vi "MenuToolOptions__slk_mt.vi"() -> ()   [LabVIEW 2020, in "Lazyboots Menu Tool.lvlib"]
uses:
  Library/Lazyboots Menu Tool.lvlib
  Private/Options/TypeDef/TypeDef_ParentSymbol__slk_mt.ctl
  Private/Options/TypeDef/TypeDef_MenuToolList__slk_mt.ctl
  Private/Options/TypeDef/TypeDef_FrameWidth__slk_mt.ctl
  Private/Options/TypeDef/TypeDef_FPGridSize.ctl
  Private/Options/TypeDef/TypeDef_ConnectorPattern__slk_mt.ctl
  Private/Options/TypeDef/TypeDef_ErrorControlStyle__slk_mt.ctl
  Private/Options/TypeDef/TypeDef_ErrorStyle__slk_mt.ctl
  Private/Options/TypeDef/TypeDef_PanelPosition__slk_mt.ctl
  Private/Options/TypeDef/TypeDef_ControlLabelPosition__slk_mt.ctl
  Private/Options/TypeDef/TypeDef_IndicatorLabelPosition__slk_mt.ctl
  Private/Options/TypeDef/TypeDef_ControlStyle__slk_mt.ctl
  Private/Options/Class/GUI/GUI__slk_mt.lvclass
  <vilib>/Utility/config.llb/NI_LVConfig.lvlib
panel:
  in  "Button: Restore":bool
  in  "Button: Cancel":bool
  in  "Button: OK":bool
  in  "Menu Tool Options":T1(tab)
  in  "Resize Panel: Ignore Decorations":bool
  in  "Resize Panel: Set Block Diagram":bool=TRUE
  in  "Resize Panel: BD Frame Width":T2=24 caption="Frame Width (pixels)"
  in  "Resize Panel: Ignore Hidden":bool=TRUE
  in  "Resize Panel: FP Position":T3="Top Left" caption="Position"
  in  "Resize Panel: FP Frame Width":T2=24 caption="Frame Width (pixels)"
  in  "Resize Panel: Set Origin":bool=TRUE
  in  "Resize Panel: Set Front Panel":bool=TRUE
  in  "Set Label Position: Apply to All":bool
  in  "Set Label Position: Indicator Label Position":T4="Right Middle" caption="Indicator Label Position"
  in  "Set Label Position: Control Label Position":T5="Left Middle" caption="Control Label Position"
  in  "Add Error: Snap to Grid":bool=TRUE
  in  "Add Error: FP Grid Size":T6=12 caption="FP Grid Size  (pixels)"
  in  "Add Error: Error Style":T7="2 Columns Style" caption="Error Style"
  in  "Add Error: Control Style":T8="Classic Style" caption="Control Style"
  in  "Add Error: Connector Pattern":T9=4815 caption="Connector Pattern" items=["4801"=4801, "4805"=4805, "4810"=4810, "4812"=4812, "4815"=4815, "4820"=4820, "4826"=4826, "4833"=4833, "4834"=4834, "4835"=4835]
  in  "Add Error: Wire to Connector":bool=TRUE
  in  "Add Error: Frame Width":T2=24 caption="Frame Width  (pixels)"
  in  "Add Error Case: Frame Width":T2=24 caption="Frame Width (pixels)"
  in  "Add Error Case: Create Constant":bool=TRUE
  in  "Create Enum: Control Style":T10="Classic Style" caption="Control Style"
  in  "Create Enum: New":bool=TRUE
  in  "Case Monitor: Parent Symbol":T11="-" caption="Parent Symbol"
  in  "Menu Tool List":T12
  # "Resize Panel"
  # "Set Label Position"
  # "Add Error"
  # "Add Error Case"
  # "Create Enum"
  # "Case Monitor"
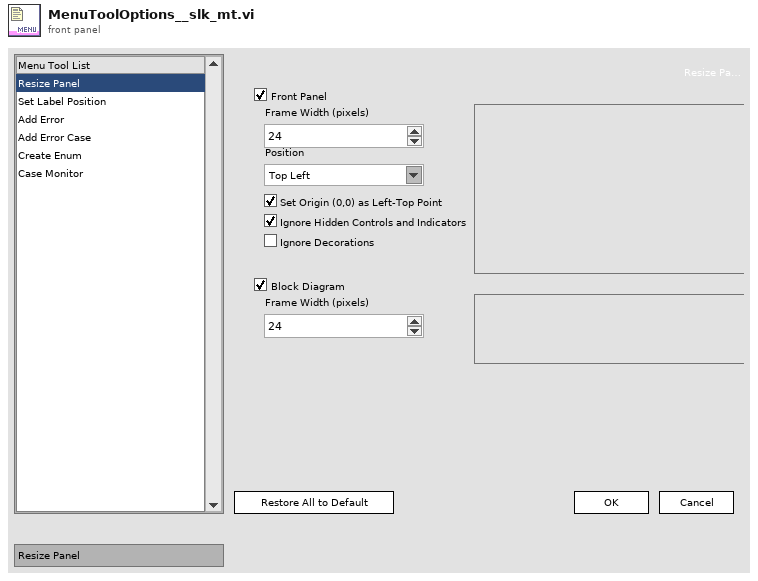
[diagram p1: front panel]
types:
  T1 = enum32{"Resize Panel", "Set Label Position", "Add Error", "Add Error Case", "Create Enum", "Case Monitor"}
  T2 = typedef "Lazyboots Menu Tool.lvlib/TypeDef_FrameWidth__slk_mt.ctl" = u32
  T3 = typedef "Lazyboots Menu Tool.lvlib/TypeDef_PanelPosition__slk_mt.ctl" = string
  T4 = typedef "Lazyboots Menu Tool.lvlib/TypeDef_IndicatorLabelPosition__slk_mt.ctl" = string
  T5 = typedef "Lazyboots Menu Tool.lvlib/TypeDef_ControlLabelPosition__slk_mt.ctl" = string
  T6 = typedef "Lazyboots Menu Tool.lvlib/TypeDef_FPGridSize.ctl" = u32
  T7 = typedef "Lazyboots Menu Tool.lvlib/TypeDef_ErrorStyle__slk_mt.ctl" = string
  T8 = typedef "Lazyboots Menu Tool.lvlib/TypeDef_ErrorControlStyle__slk_mt.ctl" = string
  T9 = typedef "Lazyboots Menu Tool.lvlib/TypeDef_ConnectorPattern__slk_mt.ctl" = u16
  T10 = typedef "Lazyboots Menu Tool.lvlib/TypeDef_ControlStyle__slk_mt.ctl" = string
  T11 = typedef "Lazyboots Menu Tool.lvlib/TypeDef_ParentSymbol__slk_mt.ctl" = string
  T12 = typedef "Lazyboots Menu Tool.lvlib/TypeDef_MenuToolList__slk_mt.ctl" = i32
  T13 = enum32{"Invalid", "Standard", "Closed", "Hidden", "Minimized", "Maximized"}
  T14 = enum8{"Enabled", "Disabled", "Disabled and Grayed Out"}
  T15 = typedef "NI_LVConfig.lvlib/Config Data RefNum.ctl" = refnum<k1>
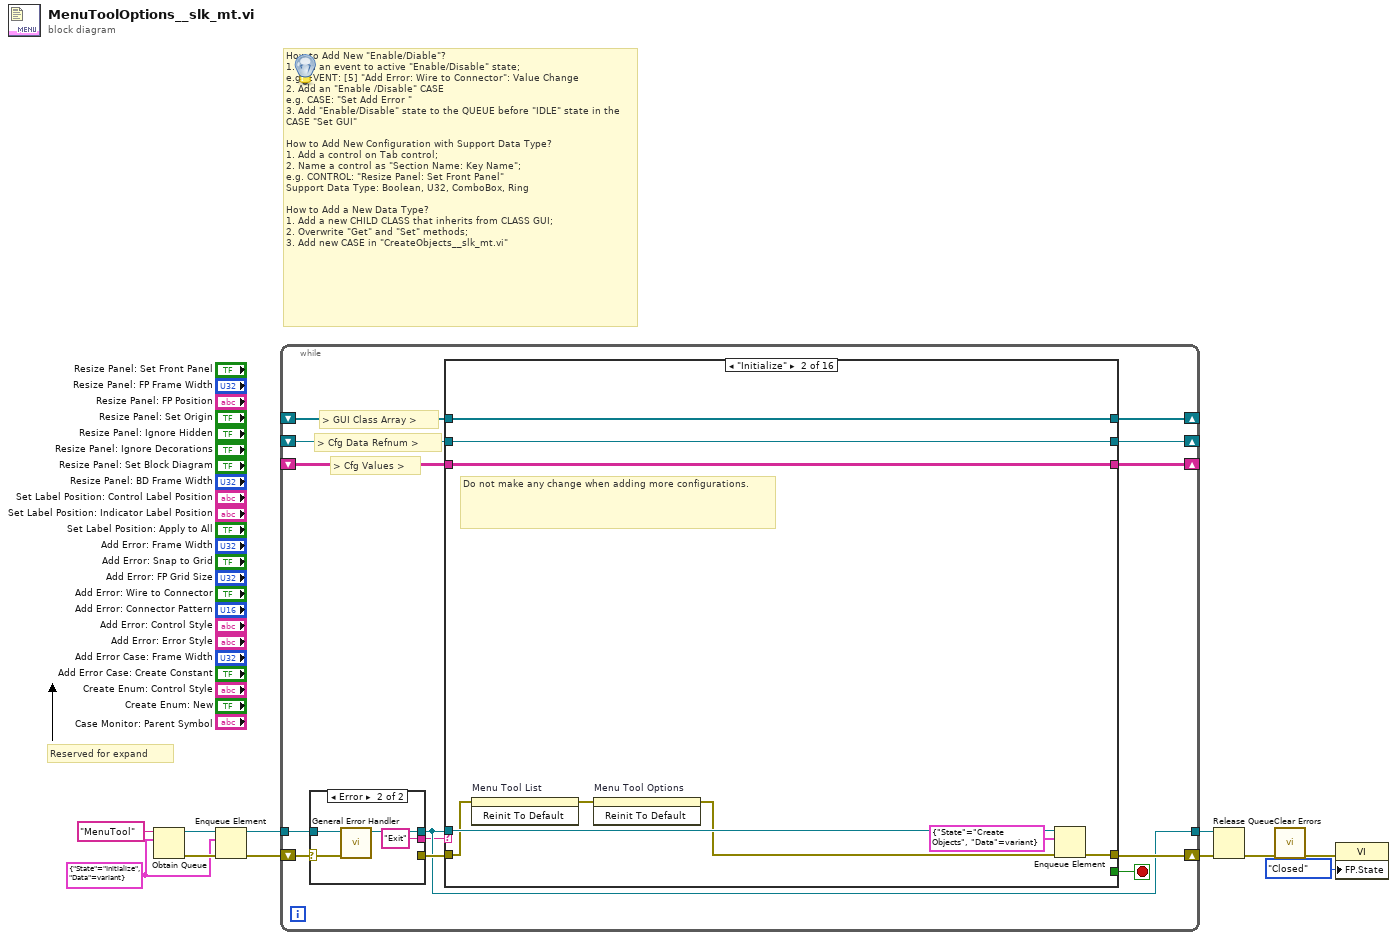
[diagram p0: block diagram]
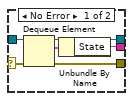
[diagram p2: hidden frame]
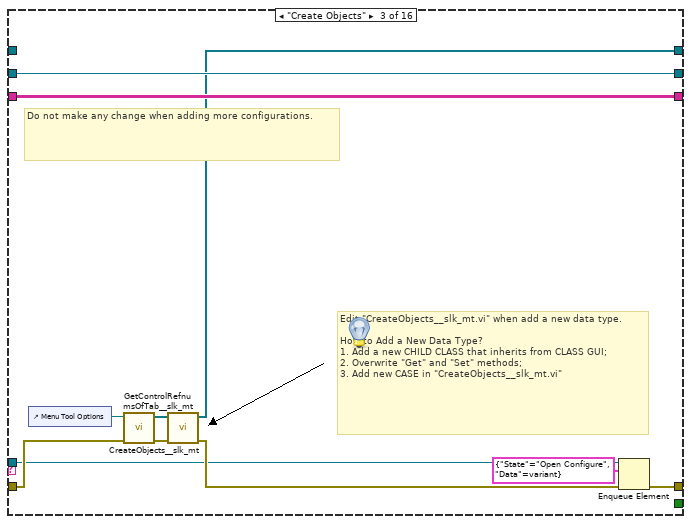
[diagram p4: hidden frame]
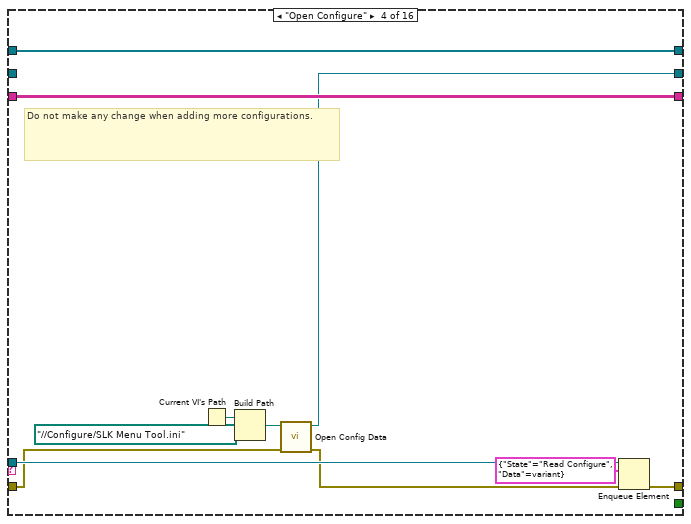
[diagram p5: hidden frame]
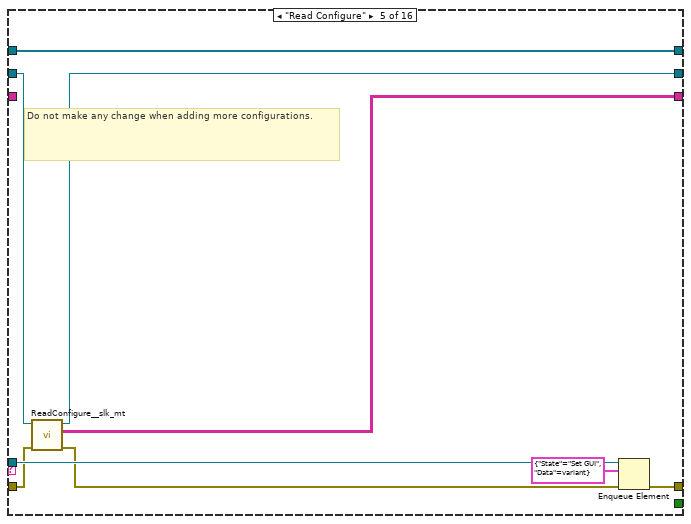
[diagram p6: hidden frame]
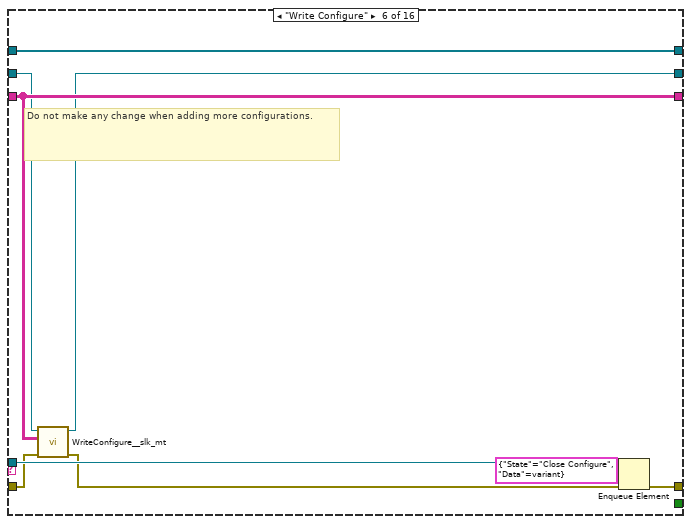
[diagram p7: hidden frame]
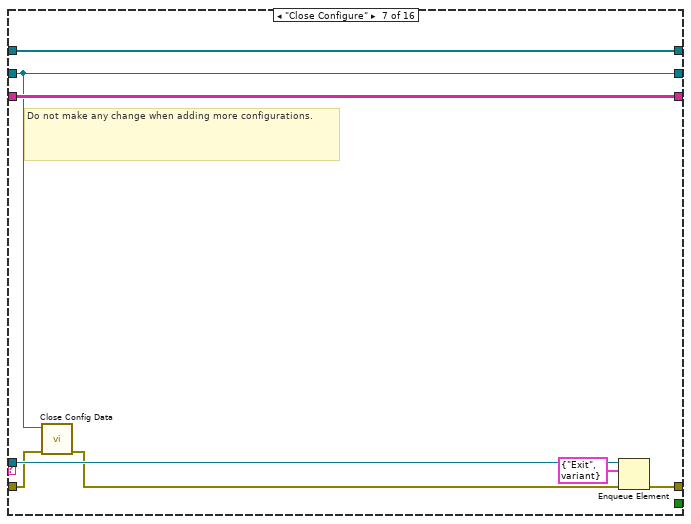
[diagram p8: hidden frame]
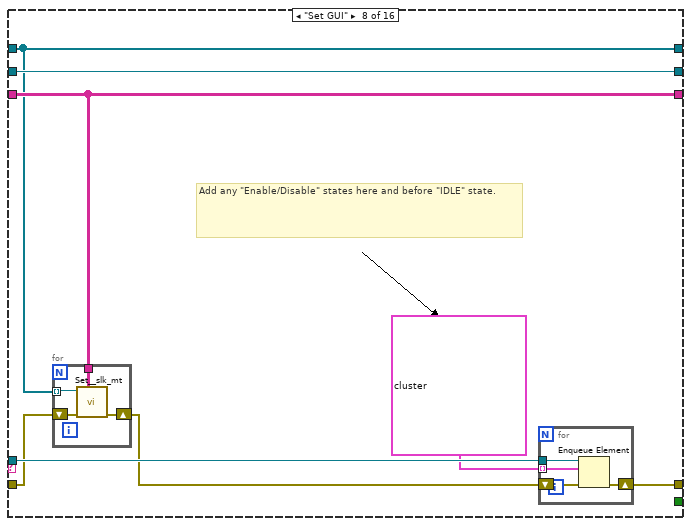
[diagram p9: hidden frame]
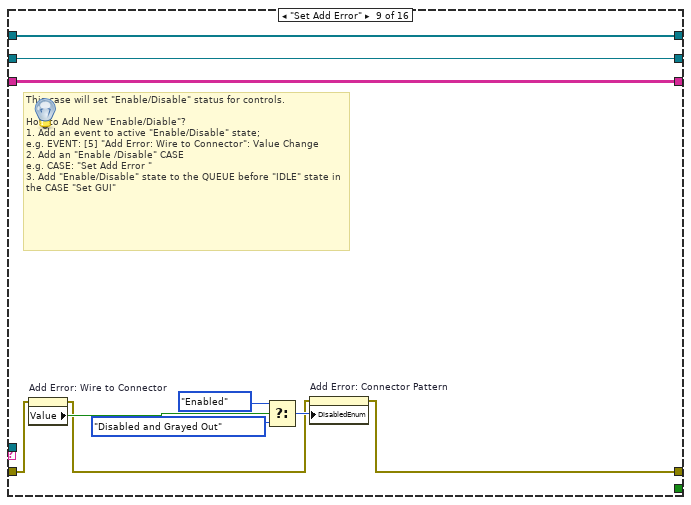
[diagram p10: hidden frame]
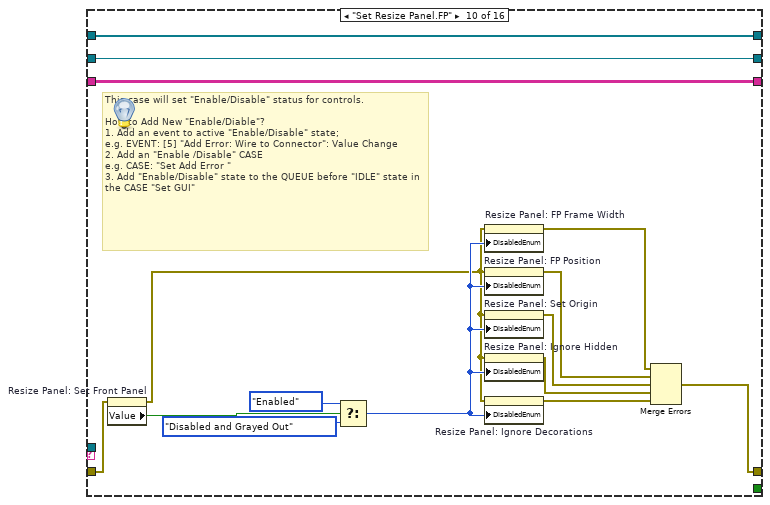
[diagram p11: hidden frame]
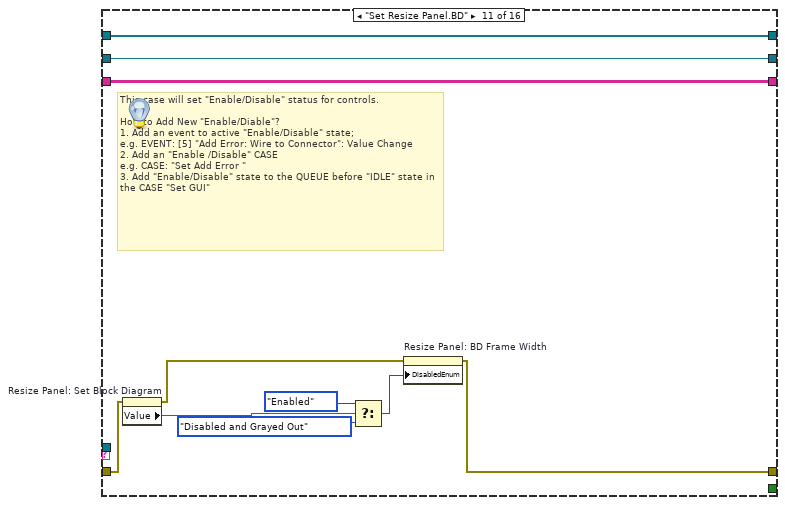
[diagram p12: hidden frame]
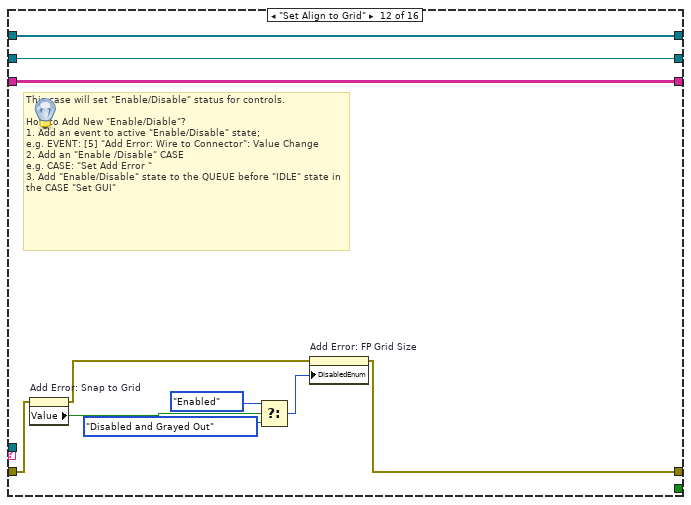
[diagram p13: hidden frame]
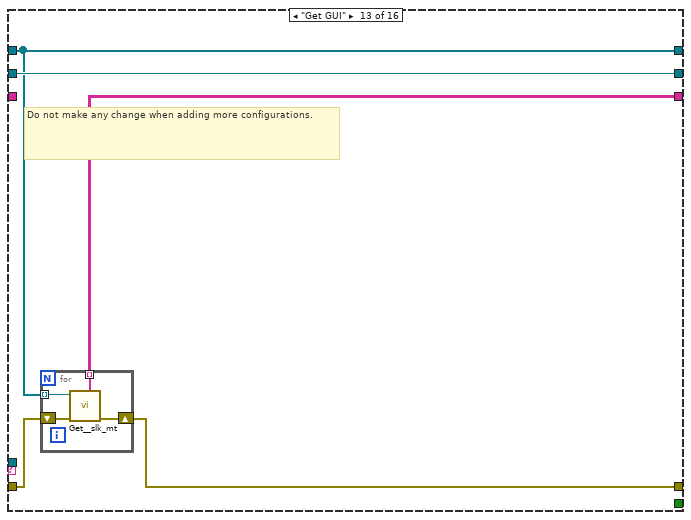
[diagram p14: hidden frame]
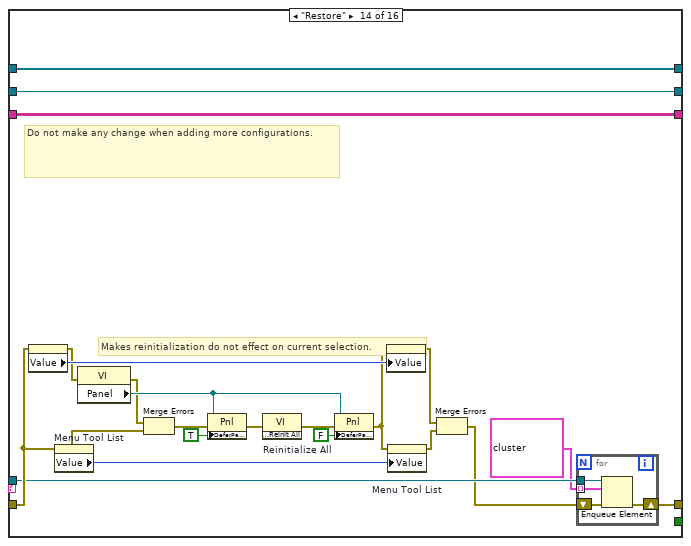
[diagram p15: hidden frame]
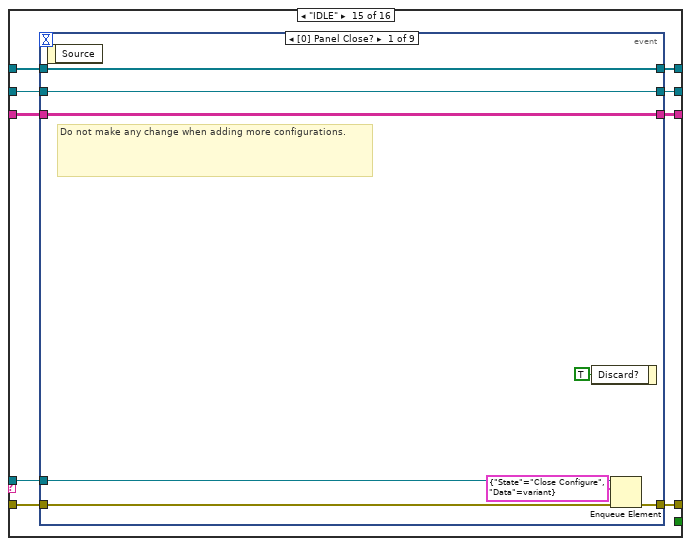
[diagram p16: hidden frame]
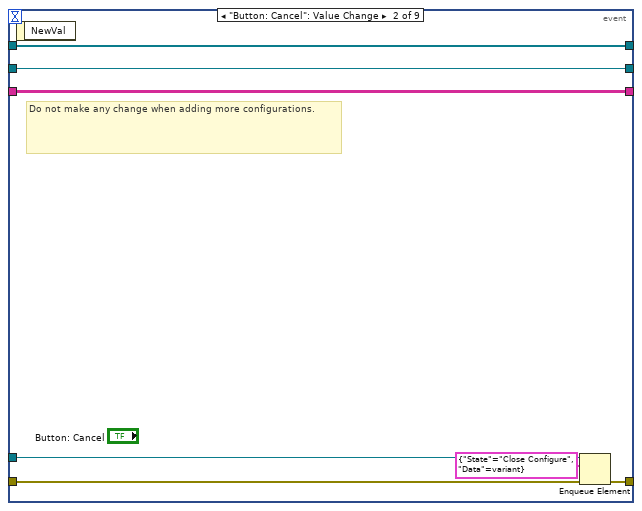
[diagram p17: hidden frame]
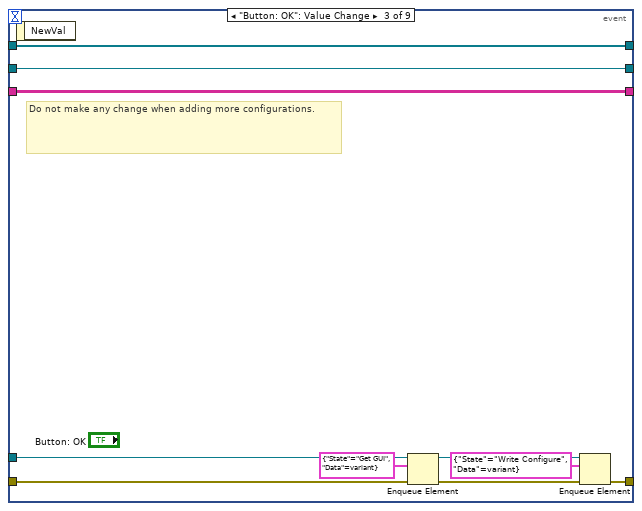
[diagram p18: hidden frame]
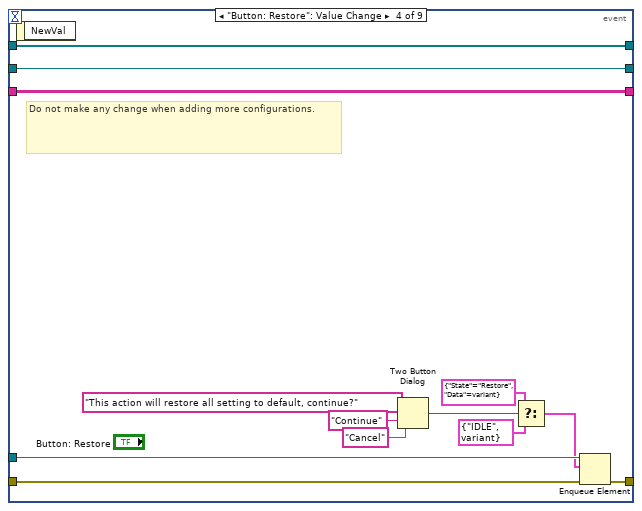
[diagram p19: hidden frame]
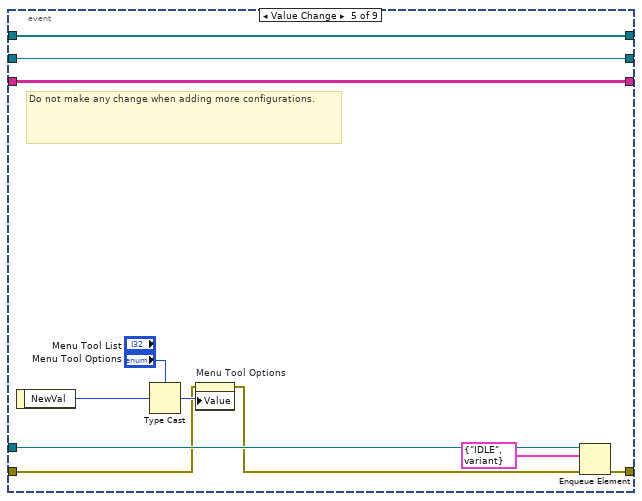
[diagram p20: hidden frame]
diagram:
  w4 = cluster{"State":string, "Data":variant} {"State"="Initialize", "Data"=variant}
  # "Reserved for expand"
  # "How to Add New \"Enable/Diable\"?\n1. Add an event to active \"Enable/Disable\" state;\ne.g. EVENT: [5] \"Add Error: Wire to Connector\": Value Change\n2. Add an \"Enable /Disable\" CASE\ne.g. CASE: \"Set Add Error \"\n3. Add \"Enable/Disable\" state to the QUEUE before \"IDLE\" state in the CASE \"Set GUI\"\n\nHow to Add New Configuration with Support Data Type?\n1. Add a control on Tab control;\n2. Name a control as \"Section Name: Key Name\";\ne.g. CONTROL: \"Resize Panel: Set Front Panel\"\nSupport Data Type: Boolean, U32, ComboBox, Ring\n\nHow to Add a New Data Type?\n1. Add a new CHILD CLASS that inherits from CLASS GUI;\n2. Overwrite \"Get\" and \"Set\" methods;\n3. Add new CASE in \"CreateObjects__slk_mt.vi\""
  n1 = Obtain Queue(name (unnamed)="MenuTool", element data type=w4) -> (queue out=w6:refnum<queue>, error out=w5:errorcluster)  [unwired: 3 in, 1 out]
  n2 = Enqueue Element(queue=w6, element=w4, error in (no error)=w5) -> (queue out=w8:refnum<queue>, error out=w9:errorcluster)  [unwired: 2 out]
  n3 = while {
    tunnel: w8 -> [w23]
    shift-right: [w21] -> w11
    shift-left: w9 -> [w24]
    shift-right: [w19] -> _
    shift-left: _ -> [w20]
    shift-right: [w15] -> _
    shift-left: _ -> [w18]
    shift-right: [w16] -> _
    shift-left: _ -> [w17]
    tunnel: [w14] -> w10
    stop <- w13 stop-if-true
    # "> Cfg Values >"
    # "> Cfg Data Refnum >"
    # "> GUI Class Array >"
    n4 = case shown="Error" w24 {
      selector: w24 -> [w29 w33]
      tunnel: w23 -> [w30 w32]
      tunnel: [w25 "Exit" ("State")] -> w12
      tunnel: [w27 _] -> w22
      tunnel: [w26 w32] -> w14
      frame No Error {
        n5 = Dequeue Element(queue=w30, error in (no error)=w29) -> (queue out=w26:refnum<queue>, element=w28:cluster{"State":string, "Data":variant}, error out=w27:errorcluster)  [unwired: 2 out]
        n6 = Unbundle By Name(w28) -> ("State"=w25:string)
      }
      frame Error {
        n7 = call <vilib>:"General Error Handler.vi"("error in (no error)"=w33) -> ()  [unwired: 2 in, 13 out]
      }
    }
    n8 = case shown="\"Initialize\"" w12 {
      tunnel: w22 -> [w37 w40 w51 w62 w70 w79 w88 w97 w112 w129 w139 w149 w157 w181 w198 w290]
      tunnel: [w37 w44 w50 w67 w77 w86 w93 w101 w111 w124 w136 w146 w156 w184 w197 w290] -> w21
      tunnel: w14 -> [_ w43 w48 w66 w76 w85 w92 w100 _ _ _ _ _ w176 w199 _]
      tunnel: w20 -> [w36 w41 _ w65 w75 w84 w91 w98 w118 w133 w143 w153 w159 w183 w196 w293]
      tunnel: [w36 w41 w53 w65 w75 w84 w91 w98 w118 w133 w143 w153 w159 w183 w195 w293] -> w19
      tunnel: w18 -> [w34 w45 w56 _ w73 w81 w89 w102 w120 w135 w145 w155 w160 w185 w194 w291]
      tunnel: w17 -> [w35 w46 w57 w68 _ w82 w94 w99 w119 w134 w144 w154 _ w186 w193 w292]
      tunnel: [w35 w46 w57 w68 w71 w82 w94 w99 w119 w134 w144 w154 w158 w186 w192 w292] -> w16
      tunnel: [w34 w45 w56 w63 w72 w80 w89 w102 w120 w135 w145 w155 w160 w185 w191 w291] -> w15
      tunnel: [_ _ _ _ _ _ _ _ _ _ _ _ _ _ _ TRUE] -> w13
      frame Default {
      }
      frame "Initialize" {
        # "Do not make any change when adding more configurations."
        n9 = invoke on="Menu Tool List" class="LstBox (strict)" method="Reinit To Default"(error in=w40) -> (error out=w39:errorcluster)  [unwired: 2 in, 2 out]
        n10 = invoke on="Menu Tool Options" class="TabCtl (strict)" method="Reinit To Default"(error in=w39) -> (error out=w38:errorcluster)  [unwired: 2 in, 2 out]
        n11 = Enqueue Element(queue=w43, element=cluster{"State":string, "Data":variant} {"State"="Create Objects", "Data"=variant}, error in (no error)=w38) -> (error out=w44:errorcluster)  [unwired: 1 in, 2 out]
      }
      frame "Create Objects" {
        # "Edit \"CreateObjects__slk_mt.vi\" when add a new data type.\n\nHow to Add a New Data Type?\n1. Add a new CHILD CLASS that inherits from CLASS GUI;\n2. Overwrite \"Get\" and \"Set\" methods;\n3. Add new CASE in \"CreateObjects__slk_mt.vi\""
        # "Do not make any change when adding more configurations."
        n12 = control-ref of="Menu Tool Options"() -> (w55:refnum<vi>)
        n13 = call "GetControlRefnumsOfTab__slk_mt.vi"("error in (no error)"=w51, "tab control refnum in"=w55) -> ("error out"=w52:errorcluster, "control refnums out"=w54:refnum<vi>[])  [unwired: 8 in]
        n14 = call "CreateObjects__slk_mt.vi"("error in (no error)"=w52, "control refnums in"=w54) -> ("error out"=w49:errorcluster, "objects out"=w53:refnum<class "GUI__slk_mt.lvclass">[])  [unwired: 8 in]
        n15 = Enqueue Element(queue=w48, element=cluster{"State":string, "Data":variant} {"State"="Open Configure", "Data"=variant}, error in (no error)=w49) -> (error out=w50:errorcluster)  [unwired: 1 in, 2 out]
      }
      frame "Open Configure" {
        # "Do not make any change when adding more configurations."
        n16 = Current VI's Path() -> (path=w58:path)
        n17 = Build Path(base path=w58, name or relative path=path "../../Configure/SLK Menu Tool.ini") -> (appended path=w60:path)
        n18 = call <vilib>:"Open Config Data.vi"("error in (no error)"=w62, "configuration file path"=w60) -> ("error out"=w61:errorcluster, "refnum"=w63:T15)  [unwired: 7 in, 1 out]
        n19 = Enqueue Element(queue=w66, element=cluster{"State":string, "Data":variant} {"State"="Read Configure", "Data"=variant}, error in (no error)=w61) -> (error out=w67:errorcluster)  [unwired: 1 in, 2 out]
      }
      frame "Read Configure" {
        # "Do not make any change when adding more configurations."
        n20 = call "ReadConfigure__slk_mt.vi"("error in (no error)"=w70, "refnum in"=w73) -> ("error out"=w69:errorcluster, "configure values"=w71:string[][], "refnum out"=w72:T15)  [unwired: 7 in]
        n21 = Enqueue Element(queue=w76, element=cluster{"State":string, "Data":variant} {"State"="Set GUI", "Data"=variant}, error in (no error)=w69) -> (error out=w77:errorcluster)  [unwired: 1 in, 2 out]
      }
      frame "Write Configure" {
        # "Do not make any change when adding more configurations."
        n22 = call "WriteConfigure__slk_mt.vi"("error in (no error)"=w79, "configure values"=w82, "refnum in"=w81) -> ("error out"=w78:errorcluster, "refnum out"=w80:T15)  [unwired: 7 in]
        n23 = Enqueue Element(queue=w85, element=cluster{"State":string, "Data":variant} {"State"="Close Configure", "Data"=variant}, error in (no error)=w78) -> (error out=w86:errorcluster)  [unwired: 1 in, 2 out]
      }
      frame "Close Configure" {
        # "Do not make any change when adding more configurations."
        n24 = call <vilib>:"Close Config Data.vi"("error in (no error)"=w88, "refnum"=w89) -> ("error out"=w87:errorcluster)  [unwired: 8 in, 1 out]
        n25 = Enqueue Element(queue=w92, element=cluster{"State":string, "Data":variant} {"State"="Exit", "Data"=variant}, error in (no error)=w87) -> (error out=w93:errorcluster)  [unwired: 1 in, 2 out]
      }
      frame "Set GUI" {
        # "Add any \"Enable/Disable\" states here and before \"IDLE\" state."
        n26 = for {
          tunnel: w99 -> [w109]
          tunnel: w98 -> [w110] mode=indexing
          shift-right: [w108] -> w96
          shift-left: w97 -> [w107]
          n27 = call-dynamic "Set__slk_mt.vi"("values"=w109, "error in (no error)"=w107, "gui in"=w110) -> ("error out"=w108:errorcluster)  [unwired: 7 in, 1 out]
        }
        n28 = for {
          tunnel: w100 -> [w105]
          shift-right: [w106] -> w101
          shift-left: w96 -> [w104]
          tunnel: cluster{"State":string, "Data":variant}[] [{"State"="Set Resize Panel.FP", "Data"=variant}, {"State"="Set Resize Panel.BD", "Data"=variant}, {"State"="Set Add Error", "Data"=variant}, {"State"="Set Align to Grid", "Data"=variant}, {"State"="IDLE", "Data"=variant}] -> [w103] mode=indexing
          n29 = Enqueue Element(queue=w105, element=w103, error in (no error)=w104) -> (error out=w106:errorcluster)  [unwired: 1 in, 2 out]
        }
      }
      frame "Set Add Error" {
        # "This case will set \"Enable/Disable\" status for controls.\n\nHow to Add New \"Enable/Diable\"?\n1. Add an event to active \"Enable/Disable\" state;\ne.g. EVENT: [5] \"Add Error: Wire to Connector\": Value Change\n2. Add an \"Enable /Disable\" CASE\ne.g. CASE: \"Set Add Error \"\n3. Add \"Enable/Disable\" state to the QUEUE before \"IDLE\" state in the CASE \"Set GUI\""
        n30 = property on="Add Error: Wire to Connector" class="Bool (strict)"(error in=w112) -> (error out=w113:errorcluster, "Value"=w114:bool)  [unwired: 1 in, 1 out]
        n31 = Select(t=T14."Enabled" ("Disabled"), s=w114, f=T14."Disabled and Grayed Out") -> (s? t:f=w116:T14)
        n32 = property on="Add Error: Connector Pattern" class="Ring (strict)"(error in=w113, "DisabledEnum"=w116) -> (error out=w111:errorcluster)  [unwired: 1 in, 1 out]
      }
      frame "Set Resize Panel.FP" {
        # "This case will set \"Enable/Disable\" status for controls.\n\nHow to Add New \"Enable/Diable\"?\n1. Add an event to active \"Enable/Disable\" state;\ne.g. EVENT: [5] \"Add Error: Wire to Connector\": Value Change\n2. Add an \"Enable /Disable\" CASE\ne.g. CASE: \"Set Add Error \"\n3. Add \"Enable/Disable\" state to the QUEUE before \"IDLE\" state in the CASE \"Set GUI\""
        n33 = property on="Resize Panel: Set Front Panel" class="Bool (strict)"(error in=w129) -> (error out=w121:errorcluster, "Value"=w130:bool)  [unwired: 1 in, 1 out]
        n34 = Select(t=T14."Enabled" ("Disabled"), s=w130, f=T14."Disabled and Grayed Out") -> (s? t:f=w122:T14)
        n35 = property on="Resize Panel: FP Frame Width" class="DigNum (strict)"(error in=w121, "DisabledEnum"=w122) -> (error out=w128:errorcluster)  [unwired: 1 in, 1 out]
        n36 = property on="Resize Panel: FP Position" class="CmbBox (strict)"(error in=w121, "DisabledEnum"=w122) -> (error out=w127:errorcluster)  [unwired: 1 in, 1 out]
        n37 = property on="Resize Panel: Set Origin" class="Bool (strict)"(error in=w121, "DisabledEnum"=w122) -> (error out=w126:errorcluster)  [unwired: 1 in, 1 out]
        n38 = property on="Resize Panel: Ignore Hidden" class="Bool (strict)"(error in=w121, "DisabledEnum"=w122) -> (error out=w125:errorcluster)  [unwired: 1 in, 1 out]
        n39 = property on="Resize Panel: Ignore Decorations" class="Bool (strict)"(error in=w121, "DisabledEnum"=w122) -> (error out=w123:errorcluster)  [unwired: 1 in, 1 out]
        n40 = Merge Errors(w128, w127, w126, w125, w123) -> (w124:errorcluster)
      }
      frame "Set Resize Panel.BD" {
        # "This case will set \"Enable/Disable\" status for controls.\n\nHow to Add New \"Enable/Diable\"?\n1. Add an event to active \"Enable/Disable\" state;\ne.g. EVENT: [5] \"Add Error: Wire to Connector\": Value Change\n2. Add an \"Enable /Disable\" CASE\ne.g. CASE: \"Set Add Error \"\n3. Add \"Enable/Disable\" state to the QUEUE before \"IDLE\" state in the CASE \"Set GUI\""
        n41 = property on="Resize Panel: Set Block Diagram" class="Bool (strict)"(error in=w139) -> (error out=w138:errorcluster, "Value"=w140:bool)  [unwired: 1 in, 1 out]
        n42 = Select(t=T14."Enabled" ("Disabled"), s=w140, f=T14."Disabled and Grayed Out") -> (s? t:f=w137:T14)
        n43 = property on="Resize Panel: BD Frame Width" class="DigNum (strict)"(error in=w138, "DisabledEnum"=w137) -> (error out=w136:errorcluster)  [unwired: 1 in, 1 out]
      }
      frame "Set Align to Grid" {
        # "This case will set \"Enable/Disable\" status for controls.\n\nHow to Add New \"Enable/Diable\"?\n1. Add an event to active \"Enable/Disable\" state;\ne.g. EVENT: [5] \"Add Error: Wire to Connector\": Value Change\n2. Add an \"Enable /Disable\" CASE\ne.g. CASE: \"Set Add Error \"\n3. Add \"Enable/Disable\" state to the QUEUE before \"IDLE\" state in the CASE \"Set GUI\""
        n44 = property on="Add Error: Snap to Grid" class="Bool (strict)"(error in=w149) -> (error out=w148:errorcluster, "Value"=w150:bool)  [unwired: 1 in, 1 out]
        n45 = Select(t=T14."Enabled" ("Disabled"), s=w150, f=T14."Disabled and Grayed Out") -> (s? t:f=w147:T14)
        n46 = property on="Add Error: FP Grid Size" class="DigNum (strict)"(error in=w148, "DisabledEnum"=w147) -> (error out=w146:errorcluster)  [unwired: 1 in, 1 out]
      }
      frame "Get GUI" {
        # "Do not make any change when adding more configurations."
        n47 = for {
          tunnel: w159 -> [w164] mode=indexing
          shift-right: [w163] -> w156
          shift-left: w157 -> [w162]
          tunnel: [w161] -> w158 mode=indexing
          n48 = call-dynamic "Get__slk_mt.vi"("error in (no error)"=w162, "gui in"=w164) -> ("error out"=w163:errorcluster, "value"=w161:string[])  [unwired: 7 in, 1 out]
        }
      }
      frame "Restore" {
        # "Makes reinitialization do not effect on current selection."
        # "Do not make any change when adding more configurations."
        n49 = property on="Menu Tool Options" class="TabCtl (strict)"(error in=w181) -> (error out=w166:errorcluster, "Value"=w178:T1)  [unwired: 1 in, 1 out]
        n50 = property on="Menu Tool List" class="LstBox (strict)"(error in=w181) -> (error out=w177:errorcluster, "Value"=w182:T12)  [unwired: 1 in, 1 out]
        n51 = property class="VI"(error in=w166) -> (error out=w165:errorcluster, "Panel"=w171:refnum<vi>)  [unwired: 1 in, 1 out]
        n52 = Merge Errors(w165, w177) -> (w168:errorcluster)
        n53 = property class="Pnl"(reference=w171, error in=w168, "DeferPanUpdts"=TRUE ("Defer Panel Updates")) -> (error out=w173:errorcluster)  [unwired: 1 out]
        n54 = invoke on="Reinitialize All" class="VI" method="Default Vals.Reinit All"(error in=w173) -> (error out=w172:errorcluster)  [unwired: 2 in, 2 out]
        n55 = property class="Pnl"(reference=w171, error in=w172, "DeferPanUpdts"=FALSE ("Defer Panel Updates")) -> (error out=w167:errorcluster)  [unwired: 1 out]
        n56 = property on="Menu Tool Options" class="TabCtl (strict)"(error in=w167, "Value"=w178) -> (error out=w179:errorcluster)  [unwired: 1 in, 1 out]
        n57 = property on="Menu Tool List" class="LstBox (strict)"(error in=w167, "Value"=w182) -> (error out=w180:errorcluster)  [unwired: 1 in, 1 out]
        n58 = Merge Errors(w179, w180) -> (w175:errorcluster)
        n59 = for {
          tunnel: w176 -> [w189]
          shift-right: [w190] -> w184
          shift-left: w175 -> [w188]
          tunnel: cluster{"State":string, "Data":variant}[] [{"State"="Get GUI", "Data"=variant}, {"State"="Set GUI", "Data"=variant}] -> [w187] mode=indexing
          n60 = Enqueue Element(queue=w189, element=w187, error in (no error)=w188) -> (error out=w190:errorcluster)  [unwired: 1 in, 2 out]
        }
      }
      frame "IDLE" {
        n61 = event shown="[0] Panel Close?" {
          selector: _ -> [_ _ _ _ _ _ _ _ _]
          dyn-events: _ -> [_ _ _ _ _ _ _ _ _]
          timeout: _ -> [_ _ _ _ _ _ _ _ _]
          tunnel: w199 -> [w202 w209 w220 w232 w244 w254 w264 w274 w284]
          tunnel: w198 -> [w203 w210 w216 w233 w239 w250 w260 w270 w280]
          tunnel: [w207 w214 w224 w237 w248 w258 w268 w278 w288] -> w197
          tunnel: w196 -> [w206 w213 w223 w236 w247 w257 w267 w277 w287]
          tunnel: [w206 w213 w223 w236 w247 w257 w267 w277 w287] -> w195
          tunnel: w194 -> [w205 w212 w222 w235 w246 w256 w266 w276 w286]
          tunnel: w193 -> [w204 w211 w221 w234 w245 w255 w265 w275 w285]
          tunnel: [w204 w211 w221 w234 w245 w255 w265 w275 w285] -> w192
          tunnel: [w205 w212 w222 w235 w246 w256 w266 w276 w286] -> w191
          event Panel Close? {
            # "Do not make any change when adding more configurations."
            n62 = event-data() -> ()  [unwired: 2 out]
            n63 = event-data("Discard?"=TRUE) -> ()  [unwired: 1 in, 1 out]
            n64 = Enqueue Element(queue=w202, element=cluster{"State":string, "Data":variant} {"State"="Close Configure", "Data"=variant}, error in (no error)=w203) -> (error out=w207:errorcluster)  [unwired: 3 out]
          }
          event "Button: Cancel": Value Change {
            # "Do not make any change when adding more configurations."
            n65 = event-data() -> ()  [unwired: 2 out]
            n66 = Enqueue Element(queue=w209, element=cluster{"State":string, "Data":variant} {"State"="Close Configure", "Data"=variant}, error in (no error)=w210) -> (error out=w214:errorcluster)  [unwired: 3 out]
          }
          event "Button: OK": Value Change {
            # "Do not make any change when adding more configurations."
            n67 = event-data() -> ()  [unwired: 2 out]
            n68 = Enqueue Element(queue=w220, element=cluster{"State":string, "Data":variant} {"State"="Get GUI", "Data"=variant}, error in (no error)=w216) -> (queue out=w218:refnum<queue>, error out=w217:errorcluster)  [unwired: 1 in, 1 out]
            n69 = Enqueue Element(queue=w218, element=cluster{"State":string, "Data":variant} {"State"="Write Configure", "Data"=variant}, error in (no error)=w217) -> (error out=w224:errorcluster)  [unwired: 3 out]
          }
          event "Button: Restore": Value Change {
            # "Do not make any change when adding more configurations."
            n70 = event-data() -> ()  [unwired: 2 out]
            n71 = Two Button Dialog(message="This action will restore all setting to default, continue?", 1:"Cancel" ("F button name (\"Cancel\")"), 2:"Continue" ("T button name (\"OK\")")) -> (T button?=w226:bool)
            n72 = Select(t=cluster{"State":string, "Data":variant} {"State"="Restore", "Data"=variant} ("element"), s=w226, f=cluster{"State":string, "Data":variant} {"State"="IDLE", "Data"=variant} ("element")) -> (s? t:f=w225:cluster{"State":string, "Data":variant})
            n73 = Enqueue Element(queue=w232, element=w225, error in (no error)=w233) -> (error out=w237:errorcluster)  [unwired: 3 out]
          }
          event Value Change {
            # "Do not make any change when adding more configurations."
            n74 = event-data() -> ("NewVal"=w242:T12)  [unwired: 1 out]
            n75 = Type Cast(type="Menu Tool Options", x=w242) -> (*(type *) &x=w240:T1)
            n76 = property on="Menu Tool Options" class="TabCtl (strict)"(error in=w239, "Value"=w240) -> (error out=w238:errorcluster)  [unwired: 1 in, 1 out]
            n77 = Enqueue Element(queue=w244, element=cluster{"State":string, "Data":variant} {"State"="IDLE", "Data"=variant}, error in (no error)=w238) -> (error out=w248:errorcluster)  [unwired: 3 out]
          }
          event "Add Error: Wire to Connector": Value Change {
            # "Back to \"IDLE\" state"
            # "\"Enable/Disable\" state"
            # "This event will active \"Enable/Disable\" and \"IDLE\" states.\n\nHow to Add New \"Enable/Diable\"?\n1. Add an event to active \"Enable/Disable\" state;\ne.g. EVENT: [5] \"Add Error: Wire to Connector\": Value Change\n2. Add an \"Enable /Disable\" CASE\ne.g. CASE: \"Set Add Error \"\n3. Add \"Enable/Disable\" state to the QUEUE before \"IDLE\" state in the CASE \"Set GUI\""
            n78 = event-data() -> ()  [unwired: 2 out]
            n79 = Enqueue Element(queue=w254, element=cluster{"State":string, "Data":variant} {"State"="Set Add Error", "Data"=variant}, error in (no error)=w250) -> (queue out=w252:refnum<queue>, error out=w251:errorcluster)  [unwired: 1 in, 1 out]
            n80 = Enqueue Element(queue=w252, element=cluster{"State":string, "Data":variant} {"State"="IDLE", "Data"=variant}, error in (no error)=w251) -> (error out=w258:errorcluster)  [unwired: 3 out]
          }
          event "Resize Panel: Set Front Panel": Value Change {
            # "This event will active \"Enable/Disable\" and \"IDLE\" states.\n\nHow to Add New \"Enable/Diable\"?\n1. Add an event to active \"Enable/Disable\" state;\ne.g. EVENT: [5] \"Add Error: Wire to Connector\": Value Change\n2. Add an \"Enable /Disable\" CASE\ne.g. CASE: \"Set Add Error \"\n3. Add \"Enable/Disable\" state to the QUEUE before \"IDLE\" state in the CASE \"Set GUI\""
            n81 = event-data() -> ()  [unwired: 2 out]
            n82 = Enqueue Element(queue=w264, element=cluster{"State":string, "Data":variant} {"State"="Set Resize Panel.FP", "Data"=variant}, error in (no error)=w260) -> (queue out=w262:refnum<queue>, error out=w261:errorcluster)  [unwired: 1 in, 1 out]
            n83 = Enqueue Element(queue=w262, element=cluster{"State":string, "Data":variant} {"State"="IDLE", "Data"=variant}, error in (no error)=w261) -> (error out=w268:errorcluster)  [unwired: 3 out]
          }
          event "Resize Panel: Set Block Diagram": Value Change {
            # "This event will active \"Enable/Disable\" and \"IDLE\" states.\n\nHow to Add New \"Enable/Diable\"?\n1. Add an event to active \"Enable/Disable\" state;\ne.g. EVENT: [5] \"Add Error: Wire to Connector\": Value Change\n2. Add an \"Enable /Disable\" CASE\ne.g. CASE: \"Set Add Error \"\n3. Add \"Enable/Disable\" state to the QUEUE before \"IDLE\" state in the CASE \"Set GUI\""
            n84 = event-data() -> ()  [unwired: 2 out]
            n85 = Enqueue Element(queue=w274, element=cluster{"State":string, "Data":variant} {"State"="Set Resize Panel.BD", "Data"=variant}, error in (no error)=w270) -> (queue out=w272:refnum<queue>, error out=w271:errorcluster)  [unwired: 1 in, 1 out]
            n86 = Enqueue Element(queue=w272, element=cluster{"State":string, "Data":variant} {"State"="IDLE", "Data"=variant}, error in (no error)=w271) -> (error out=w278:errorcluster)  [unwired: 3 out]
          }
          event "Add Error: Snap to Grid": Value Change {
            # "This event will active \"Enable/Disable\" and \"IDLE\" states.\n\nHow to Add New \"Enable/Diable\"?\n1. Add an event to active \"Enable/Disable\" state;\ne.g. EVENT: [5] \"Add Error: Wire to Connector\": Value Change\n2. Add an \"Enable /Disable\" CASE\ne.g. CASE: \"Set Add Error \"\n3. Add \"Enable/Disable\" state to the QUEUE before \"IDLE\" state in the CASE \"Set GUI\""
            n87 = event-data() -> ()  [unwired: 2 out]
            n88 = Enqueue Element(queue=w284, element=cluster{"State":string, "Data":variant} {"State"="Set Align to Grid", "Data"=variant}, error in (no error)=w280) -> (queue out=w282:refnum<queue>, error out=w281:errorcluster)  [unwired: 1 in, 1 out]
            n89 = Enqueue Element(queue=w282, element=cluster{"State":string, "Data":variant} {"State"="IDLE", "Data"=variant}, error in (no error)=w281) -> (error out=w288:errorcluster)  [unwired: 3 out]
          }
        }
      }
      frame "Exit" {
        # "Do not make any change when adding more configurations."
      }
    }
  }
  n90 = Release Queue(queue=w10, error in (no error)=w11) -> (error out=w3:errorcluster)  [unwired: 3 out]
  n91 = call <vilib>:"Clear Errors.vi"("error in (no error)"=w3) -> ("error out"=w2:errorcluster)  [unwired: 5 in, 1 out]
  n92 = property class="VI"(error in=w2, "FP.State"=T13."Closed" ("Front Panel Window:State")) -> ()  [unwired: 1 in, 2 out]
